vi "Build VI Package_vipm_lvcicd.vi"(7 "Version string(x.x.x.x)":string, 8 "error in (no error)":errorcluster, 9 "LabVIEW Version":string="19.0", 10 "vipb":path) -> (0 "error out":errorcluster, 2 "Build Output":path, 4 "New VI Package Build Spec Data":T1, 6 "Pre VI Package Build Spec Data":T1)   [LabVIEW 2014]
uses:
  <vilib>/JKI/VIPM API/command-line/support/VI Package Build Spec Data Cluster_vipm_api.ctl
  <vilib>/JKI/VIPM API/command-line/support/Version Info Cluster_vipm_api.ctl
  <vilib>/JKI/VIPM API/VIPM API_vipm_api.lvlib
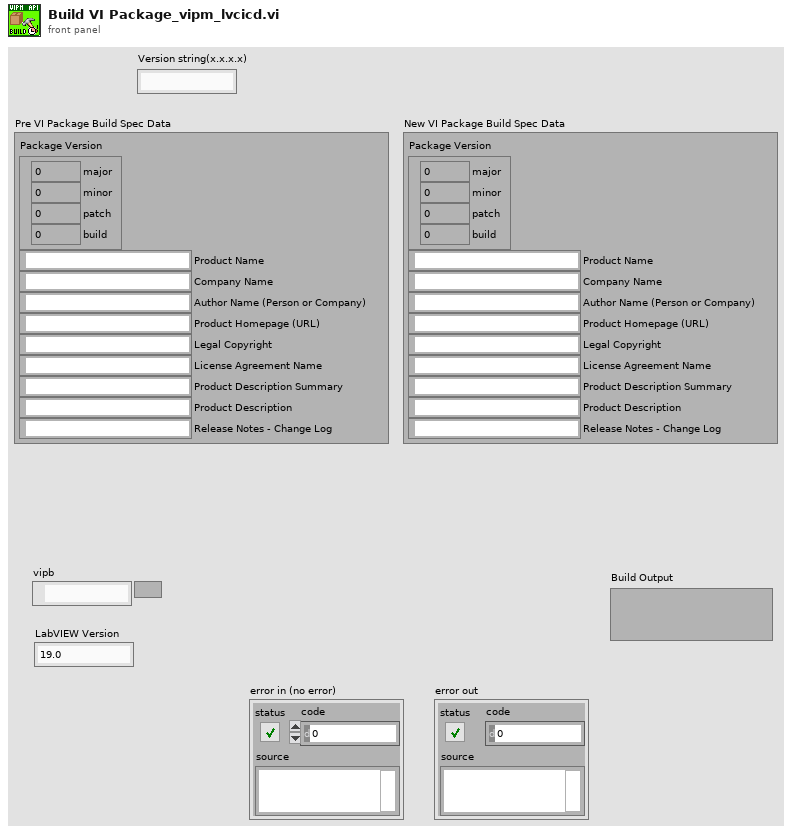
[diagram p1: front panel]
types:
  T1 = typedef "VIPM API_vipm_api.lvlib/VI Package Build Spec Data Cluster_vipm_api.ctl" = cluster{"Package Version":T2, "Product Name":string, "Company Name":string, "Author Name (Person or Company)":string, "Product Homepage (URL)":string, "Legal Copyright":string, "License Agreement Name":string, "Product Description Summary":string, "Product Description":string, "Release Notes - Change Log":string}
  T2 = typedef "VIPM API_vipm_api.lvlib/Version Info Cluster_vipm_api.ctl" = cluster{"major":u32, "minor":u32, "patch":u32, "build":u32}
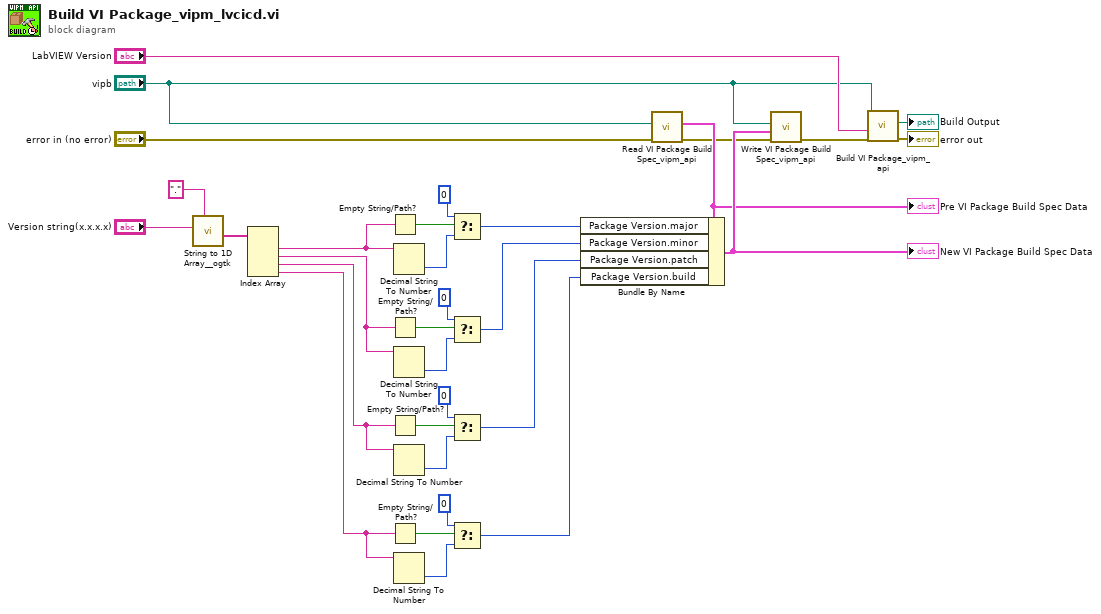
[diagram p0: block diagram]
diagram:
  n1 = call <userlib>:"String to 1D Array__ogtk.vi"("delimiter (Tab)"=".", "string"="Version string(x.x.x.x)") -> ("Array of Strings"=w21:string[])  [unwired: 9 in]
  n2 = Index Array(array=w21) -> (element #1=w18:string, element #2=w6:string, element #3=w5:string, element #4=w4:string)  [unwired: 4 in]
  n3 = Empty String/Path?(string/path=w18) -> (empty?=w20:bool)
  n4 = Empty String/Path?(string/path=w6) -> (empty?=w13:bool)
  n5 = Empty String/Path?(string/path=w5) -> (empty?=w12:bool)
  n6 = Empty String/Path?(string/path=w4) -> (empty?=w7:bool)
  n7 = Decimal String To Number(string=w18) -> (number=w17:i32)  [unwired: 2 in, 1 out]
  n8 = Decimal String To Number(string=w6) -> (number=w15:i32)  [unwired: 2 in, 1 out]
  n9 = Decimal String To Number(string=w5) -> (number=w10:i32)  [unwired: 2 in, 1 out]
  n10 = Decimal String To Number(string=w4) -> (number=w9:i32)  [unwired: 2 in, 1 out]
  n11 = Select(t=u32 0 ("Package Version.major"), s=w20, f=w17) -> (s? t:f=w16:u32)
  n12 = Select(t=u32 0 ("Package Version.major"), s=w13, f=w15) -> (s? t:f=w1:u32)
  n13 = Select(t=u32 0 ("Package Version.major"), s=w12, f=w10) -> (s? t:f=w2:u32)
  n14 = Select(t=u32 0 ("Package Version.major"), s=w7, f=w9) -> (s? t:f=w3:u32)
  n15 = call <vilib>:"Read VI Package Build Spec_vipm_api.vi"("error in (no error)"="error in (no error)", "Path to VIPB File"="vipb") -> ("error out"=w29:errorcluster, "VI Package Build Spec Data"=w30:T1)  [unwired: 8 in]
  "Pre VI Package Build Spec Data" <- w30
  n16 = Bundle By Name(cluster=w30, "Package Version.major"=w16, "Package Version.minor"=w1, "Package Version.patch"=w2, "Package Version.build"=w3) -> (w31:T1)
  "New VI Package Build Spec Data" <- w31
  n17 = call <vilib>:"Write VI Package Build Spec_vipm_api.vi"("error in (no error)"=w29, "VI Package Build Spec Data"=w31, "Path to VIPB File"="vipb") -> ("error out"=w27:errorcluster)  [unwired: 8 in]
  n18 = call <vilib>:"Build VI Package_vipm_api.vi"("error in (no error)"=w27, "LabVIEW Version"="LabVIEW Version", "Path to VIPB File"="vipb") -> ("error out"=→"error out":errorcluster, "Build Output"=→"Build Output":path)  [unwired: 7 in]
